vi "Actor Core.vi"(8 "error in":errorcluster, 11 "Grid Animation in":refnum<class "Grid Animation.lvclass">) -> (0 "error out":errorcluster, 3 "Actor out":refnum<class "Actor.lvclass">)   [LabVIEW 2024, in "Grid Animation.lvlib" / "Grid Animation.lvclass"]
doc: "<p>(<strong>Filename</strong>: <span class=\"dnl\">Actor Framework.lvlib:Actor.lvclass:Actor Core.vi</span>)</p>\n<p>Receives messages to the actor, reacts to them, and initiates any error handling that may shut the actor down.</p>\n<p>Descendant classes may override this VI to append parallel tasks for the actor to complete while it handles messages. Overrides use the <a href=\"nihelplauncher://docs/csh?context=lvcore_glang_udclass\">Call Parent Class Method</a> node.</p>"
uses:
  Grid Animation.lvclass
  C:/Program Files/National Instruments/LabVIEW 2024/vi.lib/ActorFramework/Actor/Actor.lvclass
  <vilib>/ActorFramework/Actor/Actor.lvclass
  Grid Animation.lvclass/Grid Animation.ctl
  MC Screen/Grid Screen Messages/Set Grid Value Using Coordinates Msg/Set Grid Value Using Coordinates Msg.lvclass/Set Grid Value Using Coordinates Msg.ctl
  <vilib>/ActorFramework/Message Enqueuer/Message Enqueuer.lvclass/Message Enqueuer.ctl
  <vilib>/ActorFramework/Actor/Actor.lvclass/Actor.ctl
  <vilib>/ActorFramework/Message Enqueuer/Enqueue.vi
  <vilib>/ActorFramework/Message Enqueuer/Init from Existing Queue.vi
  MC Screen/Grid Screen Messages/Set Grid Value Using Coordinates Msg/Set Grid Value Using Coordinates Msg.lvclass
  C:/Program Files/National Instruments/LabVIEW 2024/vi.lib/ActorFramework/Message/Message.lvclass
  Grid Animation Messages/Update Pattern Msg/Update Pattern Msg.lvclass
  <vilib>/ActorFramework/Message Priority Queue/Priority Enqueue.vi
  <vilib>/ActorFramework/Message Enqueuer/Message Enqueuer.lvclass
  C:/Users/ekerry/challenge-of-champions/Grid Animation/Grid Animation/Grid Animation.lvclass
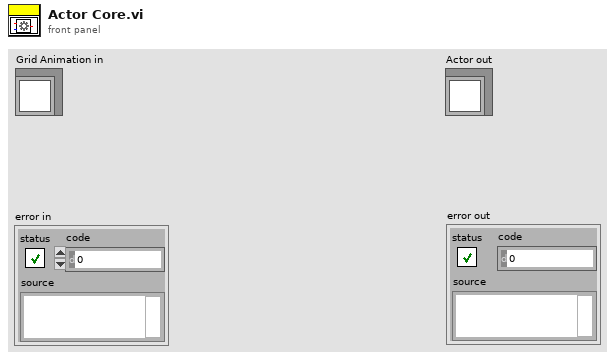
[diagram p1: front panel]
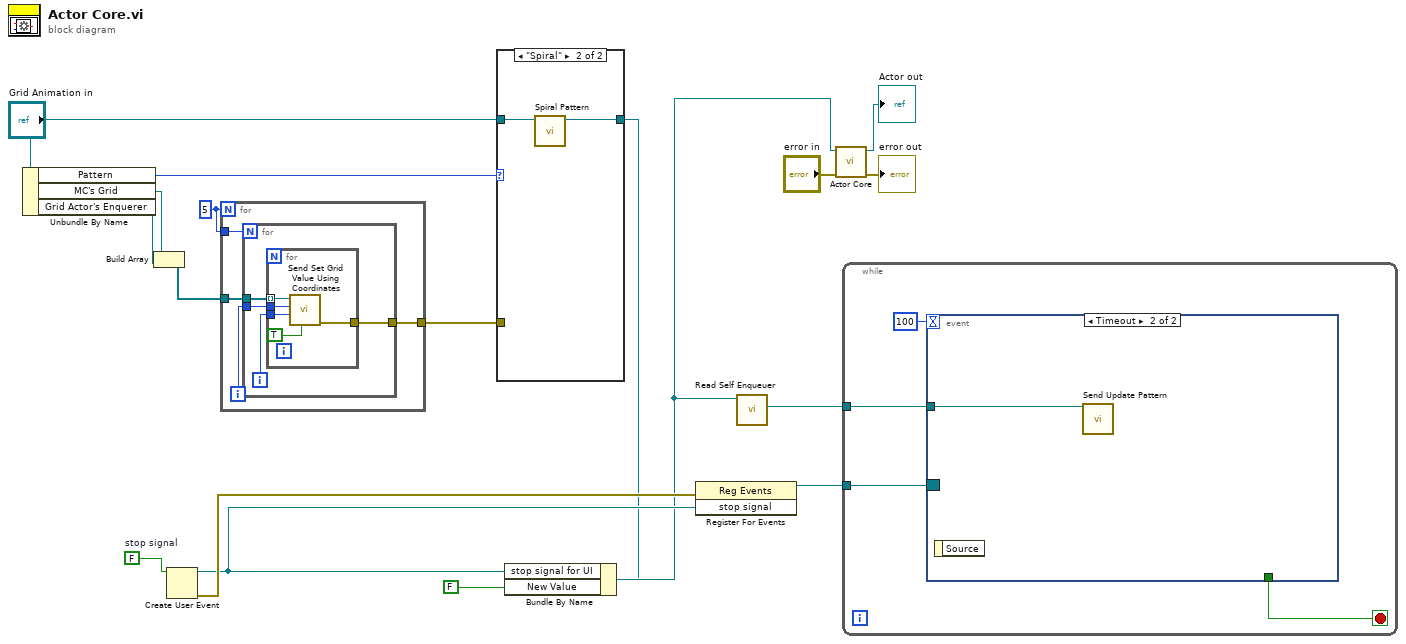
[diagram p0: block diagram]
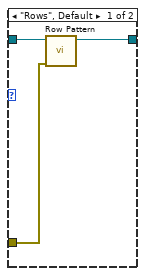
[diagram p2: hidden frame]
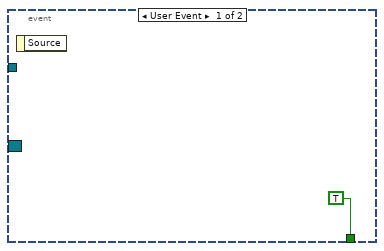
[diagram p3: hidden frame]
diagram:
  w4 = 5
  w13 = FALSE  # stop signal
  n1 = Unbundle By Name("Grid Animation in") -> ("Pattern"=w1:enum16{"Rows", "Spiral"}, "MC's Grid"=w7:refnum<class "Message Enqueuer.lvclass">, "Grid Actor's Enquerer"=w6:refnum<class "Message Enqueuer.lvclass">)
  n2 = Build Array(w7, w6) -> (w5:refnum<class "Message Enqueuer.lvclass">[])
  n3 = Create User Event(user event datatype=w13) -> (user event=w14:refnum<user-event>, error out=w15:errorcluster)  [unwired: 1 in]
  n4 = for {
    N: w4 -> [_]
    tunnel: w5 -> [w22]
    tunnel: w4 -> [w21]
    tunnel: [w19] -> w3
    i -> [w20]
    n5 = for {
      N: w21 -> [_]
      tunnel: w22 -> [w26]
      tunnel: w20 -> [w25]
      tunnel: [w23] -> w19
      i -> [w24]
      n6 = for {
        tunnel: w26 -> [w31] mode=indexing
        tunnel: w25 -> [w30]
        tunnel: w24 -> [w29]
        tunnel: [w27] -> w23
        n7 = call "Send Set Grid Value Using Coordinates.vi"("Cell Value"=TRUE, "Row"=w29, "Column"=w30, "Message Enqueuer"=w31) -> ("error out"=w27:errorcluster)  [unwired: 6 in, 1 out]
      }
    }
  }
  n8 = case shown="\"Spiral\"" w1 {
    tunnel: [w34 w35] -> w9
    tunnel: "Grid Animation in" -> [w33 w36]
    tunnel: w3 -> [w32 _]
    frame "Rows", Default {
      n9 = call-dynamic "Row Pattern.vi"("error in (no error)"=w32, "Grid Animation in"=w33) -> ("Grid Animation out"=w34:refnum<class "Grid Animation.lvclass">)  [unwired: 8 in, 1 out]
    }
    frame "Spiral" {
      n10 = call-dynamic "Spiral Pattern.vi"("Grid Animation in"=w36) -> ("Grid Animation out"=w35:refnum<class "Grid Animation.lvclass">)  [unwired: 9 in, 1 out]
    }
  }
  n11 = Bundle By Name(cluster=w9, "stop signal for UI"=w14, "New Value"=FALSE) -> (w11:refnum<class "Grid Animation.lvclass">)
  n12 = register-events(error in=w15, w14) -> (reference out=w12:refnum<event-registration>)  [unwired: 1 in, 1 out]
  n13 = call <vilib>:"Read Self Enqueuer.vi"("Actor"=w11) -> ("Self Enqueuer"=w10:refnum<class "Message Enqueuer.lvclass">)  [unwired: 10 in]
  n14 = call-parent "Actor Core.vi"("error in"="error in", "Actor in"=w11) -> ("error out"=→"error out":errorcluster, "Actor out"=→"Actor out":refnum<class "Actor.lvclass">)  [unwired: 8 in]
  n15 = while {
    tunnel: w12 -> [w39]
    tunnel: w10 -> [w37]
    stop <- w38 stop-if-true
    n16 = event shown="[1] Timeout" {
      selector: w39 -> [_ _]
      dyn-events: _ -> [_ _]
      timeout: 100 -> [_ _]
      tunnel: [TRUE _] -> w38
      tunnel: w37 -> [_ w42]
      event User Event {
        n17 = event-data() -> ()  [unwired: 1 in, 1 out]
      }
      event Timeout {
        n18 = event-data() -> ()  [unwired: 1 in, 1 out]
        n19 = call "Send Update Pattern.vi"("Message Enqueuer"=w42) -> ()  [unwired: 9 in, 2 out]
      }
    }
  }
